vi "release connections and error processor.vi"(11 "comms":T1) -> ()   [LabVIEW 2018]
uses:
  type defs/comms loop data.ctl
  ICL-LabVIEW_General/Incident logger/Incident logger.lvclass
  <vilib>/Modbus/master/Modbus Master.lvclass
  <vilib>/dex/Flush And Wait Empty Condition.ctl
  ICL-LabVIEW_General/Pulser Controller/AKD MODBUS commands/stop drive.vi
  ICL-LabVIEW_General/Pulser Controller/AKD MODBUS commands/disable drive.vi
  ICL-LabVIEW_General/Incident logger/Incidents/Quit/Quit.lvclass
  ICL-LabVIEW_General/Pulser Controller/Pulser controller commands library.lvlib
types:
  T1 = typedef "comms loop data.ctl" = cluster{"params":cluster{"commandStream":cluster{"reader name":string, "writer name":string, "stream buffer size":i32}, "errorStream":cluster{"reader name":string, "writer name":string, "stream buffer size":i32}, "RT IP address":string, "pulserControllerIP":string}, "vars":cluster{"commandStream":refnum<k21>, "Incident logger":refnum<class "Incident logger.lvclass">, "check error scheduled message":u32, "errorStream":refnum<k21>, "watchdogScheduleID":u32, "pulsator":cluster{"pulser connection":refnum<class "Modbus Master.lvclass">, "pulserConnected":bool, "pulsatorScheduleID":u32, "pulserRunning":bool}}}
  T2 = typedef "Flush And Wait Empty Condition.ctl" = u8
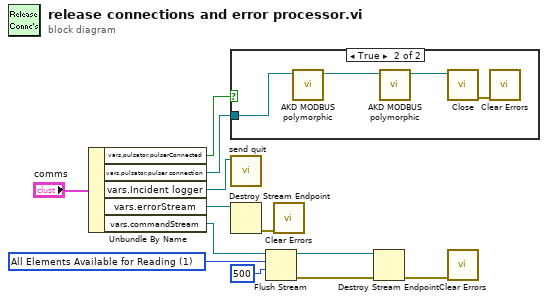
[diagram p0: block diagram]
diagram:
  w6 = T2 1 items=["All Elements Read From Stream", "All Elements Available for Reading"] ("wait condition")
  n1 = Unbundle By Name("comms") -> ("vars.pulsator.pulserConnected"=w2:bool, "vars.pulsator.pulser connection"=w1:refnum<class "Modbus Master.lvclass">, "vars.Incident logger"=w12:refnum<class "Incident logger.lvclass">, "vars.errorStream"=w10:refnum<k21>, "vars.commandStream"=w7:refnum<k21>)
  n2 = case shown="True" w2 {
    tunnel: w1 -> [_ w15]
    frame False {
    }
    frame True {
      n3 = call-poly "AKD MODBUS polymorphic.vi"("Modbus Master in"=w15) -> ("Modbus Master out"=w14:refnum<class "Modbus Master.lvclass">)  [unwired: 10 in]
      n4 = call-poly "AKD MODBUS polymorphic.vi"("Modbus Master in"=w14) -> ("Modbus Master out"=w13:refnum<class "Modbus Master.lvclass">)  [unwired: 10 in]
      n5 = call-dynamic "Close.vi"("Modbus master in"=w13) -> ("error out"=w16:errorcluster)  [unwired: 10 in]
      n6 = call <vilib>:"Clear Errors.vi"("error in (no error)"=w16) -> ()  [unwired: 5 in, 2 out]
    }
  }
  n7 = call "send quit.vi"("incident logger"=w12) -> ()  [unwired: 10 in, 1 out]
  n8 = Destroy Stream Endpoint(11:w10) -> (0:w8:errorcluster)  [unwired: 1 in]
  n9 = Flush Stream(9:500 ("timeout in ms (-1)"), 10:w6, 11:w7) -> (0:w3:errorcluster, 3:w5:refnum<k21>)  [unwired: 1 in, 1 out]
  n10 = call <vilib>:"Clear Errors.vi"("error in (no error)"=w8) -> ()  [unwired: 5 in, 2 out]
  n11 = Destroy Stream Endpoint(8:w3, 11:w5) -> (0:w9:errorcluster)
  n12 = call <vilib>:"Clear Errors.vi"("error in (no error)"=w9) -> ()  [unwired: 5 in, 2 out]
